vi "Create Key Edge Map.vi"(8 "error in (no error)":errorcluster, 10 "Rising Edge?":refnum<class "1D Array binary.lvclass">, 11 "Key Map Primitive":refnum<class "2D Array u32.lvclass">) -> (0 "error out":errorcluster, 3 "Key Edge Map":refnum<class "1D Array s64.lvclass">)   [LabVIEW 2020, in "G2CPU Line Profile.lvlib"]
uses:
  G2CPU Line Profile.lvlib
  <vilib>/Natan Biesmans/G2CPU GPU and CPU HPC Toolkit/G2CPU Libraries/Arrays/1DArray/s64/1D Array s64.lvclass
  C:/Program Files/National Instruments/LabVIEW 2025/vi.lib/Natan Biesmans/G2CPU GPU and CPU HPC Toolkit/G2CPU Libraries/Arrays/Array/Array Prototype.lvclass
  <vilib>/Natan Biesmans/G2CPU GPU and CPU HPC Toolkit/G2CPU Libraries/Arrays/2DArray/u32/2D Array u32.lvclass
  <vilib>/Natan Biesmans/G2CPU GPU and CPU HPC Toolkit/G2CPU Libraries/Arrays/1DArray/binary/1D Array binary.lvclass
  <vilib>/Natan Biesmans/G2CPU GPU and CPU HPC Toolkit/G2CPU Libraries/Arrays/Array/Array Prototype.lvclass/Array Prototype.ctl
  bc61aa56-81d4-4ed7-a508-a2ff18d114bb.vi
  f44035e1-4581-4d4d-8fa9-b8d140b1495f.vi
  a79b6380-befc-4334-9246-1fe34c579cb3.vi
  79b2e88c-c1e1-4b87-9a75-dc94f8cd7df6.vi
  e8dcf560-1b77-456d-bae3-305158a98e40.vi
  38415fb8-e4a0-4506-be29-c071657200f6.vi
  fcc5b371-5cdb-49ca-b48c-bcc0f05f0908.vi
  bc61aa56-81d4-4ed7-a508-a2ff18d114bb.vi/cfed8f62-9c64-4dab-912e-5e7c21cb720b.vi
  f44035e1-4581-4d4d-8fa9-b8d140b1495f.vi/cfed8f62-9c64-4dab-912e-5e7c21cb720b.vi
  <vilib>/Natan Biesmans/G2CPU GPU and CPU HPC Toolkit/G2CPU Libraries/Arrays/Array/G2CPU Get Array Pointer.vi
  a79b6380-befc-4334-9246-1fe34c579cb3.vi/d8f9d983-4edf-44a2-8364-f00f0b470774.vi
  a79b6380-befc-4334-9246-1fe34c579cb3.vi/83167447-a0f5-45d9-a71d-4def8f50970d.vi
  79b2e88c-c1e1-4b87-9a75-dc94f8cd7df6.vi/e7247370-a01f-465a-ac0e-4dfefcb1bb87.vi
  79b2e88c-c1e1-4b87-9a75-dc94f8cd7df6.vi/345e91f0-9a5e-4de4-af9c-133346717e4a.vi
  e8dcf560-1b77-456d-bae3-305158a98e40.vi/5793b77b-c002-4ebf-9075-685617c95341.vi
  e8dcf560-1b77-456d-bae3-305158a98e40.vi/2ed3ef86-c00d-4d71-b84c-20267a6dfcf9.vi
  38415fb8-e4a0-4506-be29-c071657200f6.vi/e9bebd79-1c27-4fc1-b91f-30516104c7f0.vi
  fcc5b371-5cdb-49ca-b48c-bcc0f05f0908.vi/7467a0f1-0650-4e63-b635-b3d2b2ec9a4e.vi
  fcc5b371-5cdb-49ca-b48c-bcc0f05f0908.vi/8ee11bc3-5ef5-497e-97f0-8db2b3aaa149.vi
  fcc5b371-5cdb-49ca-b48c-bcc0f05f0908.vi/c7af9698-5e3c-4e11-95da-3024075b67d2.vi
  bc61aa56-81d4-4ed7-a508-a2ff18d114bb.vi/cfed8f62-9c64-4dab-912e-5e7c21cb720b.vi/77c7badc-ed81-4514-99c1-20d37f4e5ecc.vi
  bc61aa56-81d4-4ed7-a508-a2ff18d114bb.vi/cfed8f62-9c64-4dab-912e-5e7c21cb720b.vi/eb76fa01-6782-47b4-b34f-9eb474c9cc78.vi
  <vilib>/Natan Biesmans/G2CPU GPU and CPU HPC Toolkit/ArrayFire Driver/VIs/Run as Multi Device.vi
  f44035e1-4581-4d4d-8fa9-b8d140b1495f.vi/cfed8f62-9c64-4dab-912e-5e7c21cb720b.vi/77c7badc-ed81-4514-99c1-20d37f4e5ecc.vi
  f44035e1-4581-4d4d-8fa9-b8d140b1495f.vi/cfed8f62-9c64-4dab-912e-5e7c21cb720b.vi/eb76fa01-6782-47b4-b34f-9eb474c9cc78.vi
  e8dcf560-1b77-456d-bae3-305158a98e40.vi/5793b77b-c002-4ebf-9075-685617c95341.vi/3e802c67-fb96-46a3-ae13-4994a8508b4f.vi
  e8dcf560-1b77-456d-bae3-305158a98e40.vi/5793b77b-c002-4ebf-9075-685617c95341.vi/5a50fc67-79e7-4972-80c2-92243cd53dd4.vi
  e8dcf560-1b77-456d-bae3-305158a98e40.vi/2ed3ef86-c00d-4d71-b84c-20267a6dfcf9.vi/730f6c57-5c0b-4ee9-b61e-75067b25222b.vi
  e8dcf560-1b77-456d-bae3-305158a98e40.vi/2ed3ef86-c00d-4d71-b84c-20267a6dfcf9.vi/096b8799-7810-404e-baca-ba9279cec4bd.vi
  e8dcf560-1b77-456d-bae3-305158a98e40.vi/2ed3ef86-c00d-4d71-b84c-20267a6dfcf9.vi/0f1a5a47-bcc5-4796-ac31-8dfcfbc0d7d1.vi
  e8dcf560-1b77-456d-bae3-305158a98e40.vi/2ed3ef86-c00d-4d71-b84c-20267a6dfcf9.vi/89f12e17-3330-4b72-ad8f-8dd636660732.vi
  <vilib>/Natan Biesmans/G2CPU GPU and CPU HPC Toolkit/G2CPU Libraries/Arrays/2DArray/s64/2D Array s64.lvclass
  <vilib>/Natan Biesmans/G2CPU GPU and CPU HPC Toolkit/ArrayFire Driver/VIs/iszero.vi
  <vilib>/Natan Biesmans/G2CPU GPU and CPU HPC Toolkit/ArrayFire Driver/VIs/sub.vi
  <vilib>/Natan Biesmans/G2CPU GPU and CPU HPC Toolkit/ArrayFire Driver/VIs/release array.vi
  <vilib>/Natan Biesmans/G2CPU GPU and CPU HPC Toolkit/ArrayFire Driver/subvi/Error Converter (ErrCode or Status).vi
  <vilib>/Natan Biesmans/G2CPU GPU and CPU HPC Toolkit/ArrayFire Driver/VIs/cast.vi
  <vilib>/Natan Biesmans/G2CPU GPU and CPU HPC Toolkit/ArrayFire Driver/VIs/add.vi
  <vilib>/Natan Biesmans/G2CPU GPU and CPU HPC Toolkit/G2CPU Libraries/Arrays/Array/G2CPU Set Array Pointer.vi
  <vilib>/Natan Biesmans/G2CPU GPU and CPU HPC Toolkit/ArrayFire Driver/VIs/replace.vi
  <vilib>/Natan Biesmans/G2CPU GPU and CPU HPC Toolkit/G2CPU Libraries/Arrays/Array/G2CPU Release Array.vi
  <vilib>/Natan Biesmans/G2CPU GPU and CPU HPC Toolkit/G2CPU Libraries/Arrays/SubVI/is 2D.vi
  <vilib>/Natan Biesmans/G2CPU GPU and CPU HPC Toolkit/ArrayFire Driver/VIs/transpose.vi
  <vilib>/Natan Biesmans/G2CPU GPU and CPU HPC Toolkit/ArrayFire Driver/VIs/flat.vi
  <vilib>/Natan Biesmans/G2CPU GPU and CPU HPC Toolkit/G2CPU Libraries/Arrays/1DArray/1D Array Prototype.lvclass
  <vilib>/Natan Biesmans/G2CPU GPU and CPU HPC Toolkit/G2CPU Libraries/Arrays/Array/Array Prototype.lvclass
  <vilib>/Natan Biesmans/G2CPU GPU and CPU HPC Toolkit/G2CPU Libraries/Arrays/2DArray/2D Array Prototype.lvclass
  <vilib>/Natan Biesmans/G2CPU GPU and CPU HPC Toolkit/G2CPU Libraries/Arrays/DataTypes/I64/s64.lvclass
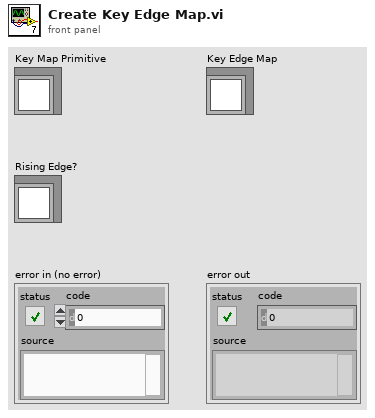
[diagram p1: front panel]
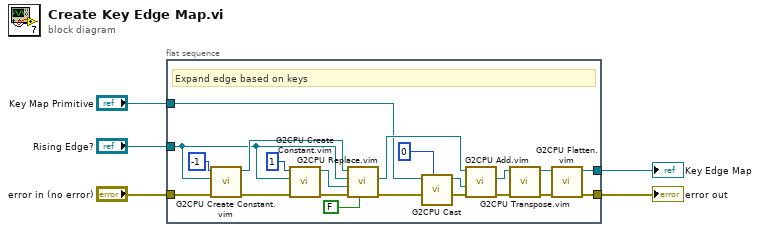
[diagram p0: block diagram]
diagram:
  n1 = flat-sequence {
    tunnel: "Rising Edge?" -> [w16]
    tunnel: "Key Map Primitive" -> [w11]
    tunnel: "error in (no error)" -> [w10]
    tunnel: [w8] -> w4
    tunnel: [w7] -> w5
    frame #0 {
      # "Expand edge based on keys"
      n2 = call "G2CPU Create Constant.vim"("error in (no error)"=w10, "Size"=w16, "val"=i64 -1) -> ("error out"=w19:errorcluster, "object out"=w18:refnum<class "1D Array s64.lvclass">)  [unwired: 7 in]
      n3 = call "G2CPU Create Constant.vim"("error in (no error)"=w19, "Size"=w16, "val"=i64 1) -> ("error out"=w15:errorcluster, "object out"=w17:refnum<class "1D Array s64.lvclass">)  [unwired: 7 in]
      n4 = call "G2CPU Replace.vim"("Auto Release Replace Condition (Enabled)"=FALSE, "error in (no error)"=w15, "To Replace Values Array or scalar Value"=w17, "Replace  Condition"=w16, "Array In"=w18) -> ("error out"=w14:errorcluster, "Array out (same as in)"=w12:refnum<class "1D Array s64.lvclass">)  [unwired: 5 in]
      n5 = call "G2CPU Cast"("Datatype Prototype"=i64 0 ("val"), "error in (no error)"=w14, "Array In"=w11) -> ("error out"=w22:errorcluster, "Array Out"=w13:refnum<class "2D Array s64.lvclass">)  [unwired: 7 in]
      n6 = call "G2CPU Add.vim"("error in (no error)"=w22, "Array rhs"=w13, "Array lhs"=w12) -> ("error out"=w24:errorcluster, "Array Result"=w23:refnum<class "2D Array s64.lvclass">)  [unwired: 7 in]
      n7 = call "G2CPU Transpose.vim"("error in (no error)"=w24, "Array In"=w23) -> ("error out"=w26:errorcluster, "Array out"=w25:refnum<class "2D Array s64.lvclass">)  [unwired: 8 in]
      n8 = call "G2CPU Flatten.vim"("error in (no error)"=w26, "Array In"=w25) -> ("error out"=w8:errorcluster, "Array out"=w7:refnum<class "1D Array s64.lvclass">)  [unwired: 8 in]
    }
  }
  "Key Edge Map" <- w5
  "error out" <- w4
